vi "Accessories.vi"(11 "Full System Configuration":T2={"Rack"=enum."15U; 1-Phase; 16A; 100-240V", "Middle Rail"=enum."None", "Ballast"={"Main"=0, "Small"=0, "Side"=0}, "Front Panel I/O"={"EMO Button"=FALSE, "USB 3.0"=FALSE, "Display"=FALSE, "1st USB 2.0"=FALSE, "2nd USB 2.0"=FALSE, "Ethernet 3"=FALSE, "EMO Extension (3rd Party)"=FALSE, "EMO Extension (Rack In & Out)"=FALSE, "Aux Dual C13 QAC Outlets"=FALSE, "Residual-current Circuit Breaker"=FALSE, "Serial"=FALSE, "GPIB"=FALSE}, "Rear Panel I/O"={"Rear Panel I/O Configuration"=enum."Blank Panel", "EMO Button"=FALSE, "Power, Status & Banana Ground"=FALSE, "Ethernet 2"=FALSE, "Display"=FALSE, "USB 3.0"=FALSE, "DIO"=FALSE, "GPIB"=FALSE, "Aux Dual C13 QAC Outlets"=FALSE, "Residual-current Circuit Breaker"=FALSE, "Serial"=FALSE, "SMA"=FALSE}, "Miscellaneous Options"={"Eyebolts"=FALSE, "Tower Light"=FALSE, "Top/Side Monitor Mount Kit"=FALSE, "24\" Monitor"=FALSE, "Keyboard & Mouse"=FALSE, "Secondary Ethernet Switch"=FALSE, "Extra USB Hub"=FALSE, "USB-6509"=FALSE, "Front Door"=enum."38U (Solid) IG", "Primary Ethernet Switch"=enum."Item 0", "Use Posture"=enum."Item 0"}, "Accessories"={"Screw Type"=enum."10-32", "Cage Nuts & Screws"=0.0, "Filler Panel Color"=enum."Interface Gray", "1U"=0.0, "2U"=0.0, "3U"=0.0}} {"Ballast"."Side" max=5 step=1; "Ballast"."Small" max=5 step=1; "Ballast"."Main" max=5 step=1}) -> (3 "Accessories Out":T1[](array[typedef]))   [LabVIEW 2023]
uses:
  Option Type Defs/Full System Configuration.ctl
  Option Type Defs/Rack.ctl
  Option Type Defs/Middle Rail.ctl
  Option Type Defs/Ballast.ctl
  Option Type Defs/Front Panel IO.ctl
  Option Type Defs/Rear Panel IO.ctl
  Option Type Defs/Rear Panel IO Configuration.ctl
  Option Type Defs/Miscellaneous Options.ctl
  Option Type Defs/Front Door.ctl
  Option Type Defs/Accessories.ctl
  Option Type Defs/Screw Types.ctl
  Option Type Defs/Filler Panel Color.ctl
  Option Type Defs/Parts List.ctl
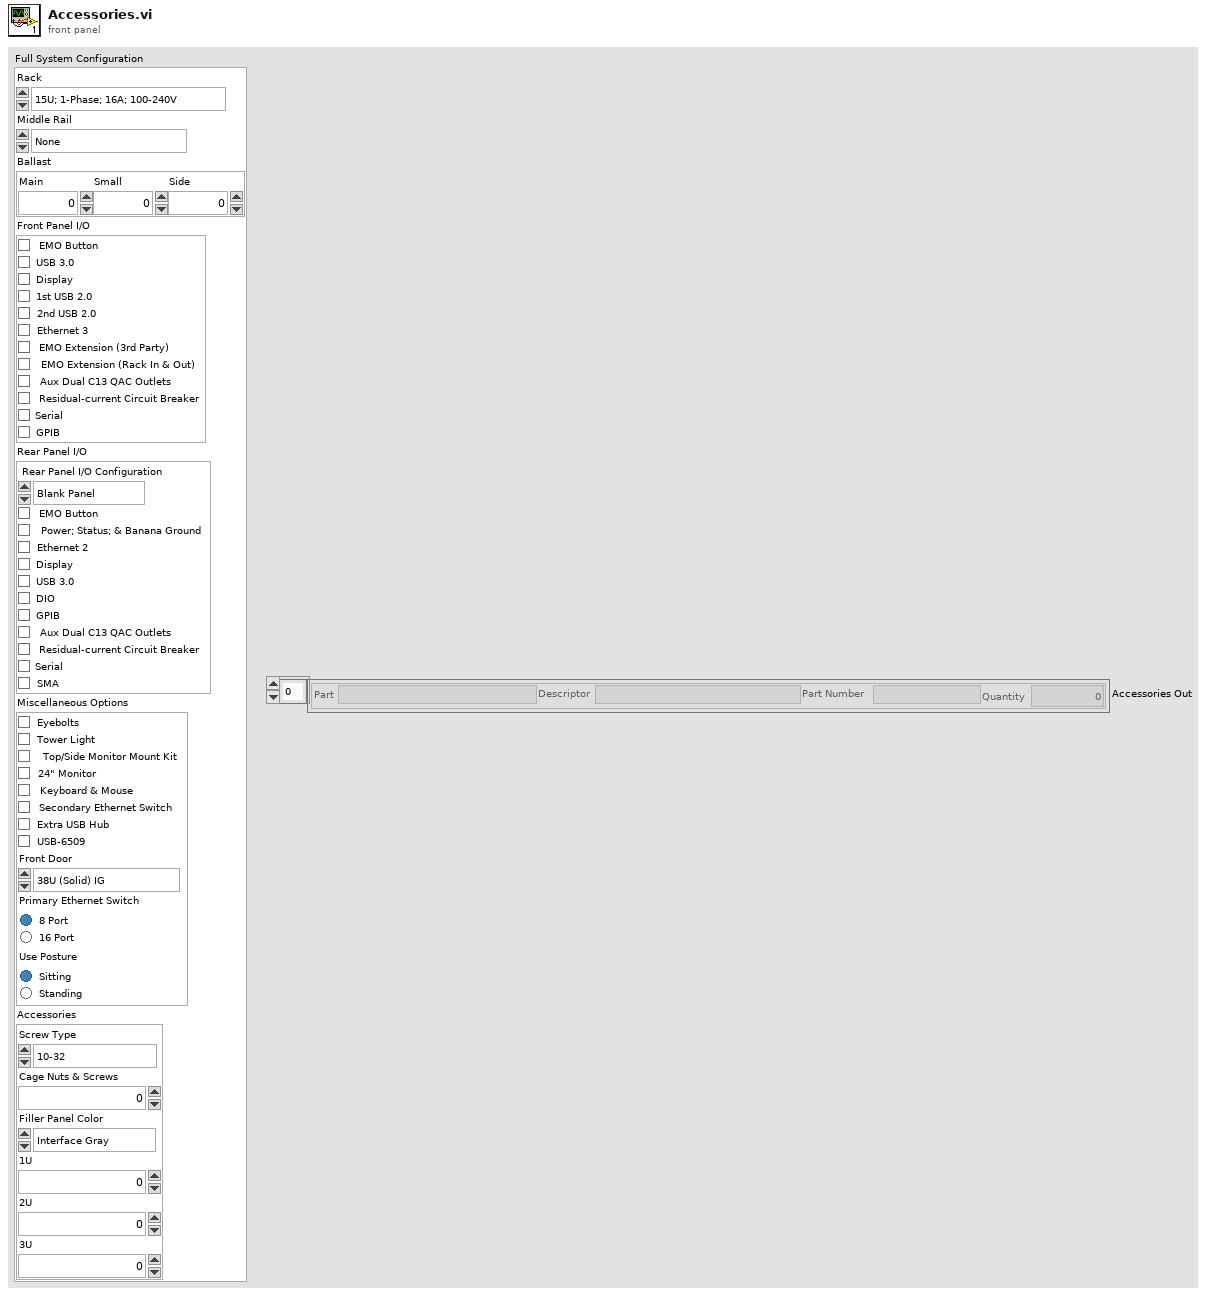
[diagram p1: front panel]
types:
  T1 = typedef "Parts List.ctl" = cluster{"Part":string, "Descriptor":string, "Part Number":string, "Quantity":dbl}
  T2 = typedef "Full System Configuration.ctl" = cluster{"Rack":T3, "Middle Rail":T4, "Ballast":T5, "Front Panel I/O":T6, "Rear Panel I/O":T7, "Miscellaneous Options":T9, "Accessories":T11}
  T3 = typedef "Rack.ctl" = enum16{"15U; 1-Phase; 16A; 100-240V", "15U; 1-Phase; 24A; 100-240V", "38U; 3-Phase Delta; 50A; 200-240V", "38U; 1-Phase; 24A; 100-120V", "38U; 3-Phase Wye; 50A; 200-240V", "38U; 3-Phase Delta; 50A; 380-480V", "38U; 3-Phase Delta; 32A; 200-240V", "38U; 3-Phase Wye; 16A; 100-240V", "44U; 1-Phase; 24A; 100-240V", "44U; 3-Phase Delta; 32A; 200-240V"}
  T4 = typedef "Middle Rail.ctl" = enum16{"None", "Flip Side Rear; D=168.83mm", "Parallel Rear; D=145mm", "Flip Side Front; D=145mm", "Parallel Front; D=145mm"}
  T5 = typedef "Ballast.ctl" = cluster{"Main":u16, "Small":u16, "Side":u16}
  T6 = typedef "Front Panel IO.ctl" = cluster{"EMO Button":bool, "USB 3.0":bool, "Display":bool, "1st USB 2.0":bool, "2nd USB 2.0":bool, "Ethernet 3":bool, "EMO Extension (3rd Party)":bool, "EMO Extension (Rack In & Out)":bool, "Aux Dual C13 QAC Outlets":bool, "Residual-current Circuit Breaker":bool, "Serial":bool, "GPIB":bool}
  T7 = typedef "Rear Panel IO.ctl" = cluster{"Rear Panel I/O Configuration":T8, "EMO Button":bool, "Power, Status & Banana Ground":bool, "Ethernet 2":bool, "Display":bool, "USB 3.0":bool, "DIO":bool, "GPIB":bool, "Aux Dual C13 QAC Outlets":bool, "Residual-current Circuit Breaker":bool, "Serial":bool, "SMA":bool}
  T8 = typedef "Rear Panel IO Configuration.ctl" = enum16{"Blank Panel", "Fully Populated Panel", "Custom Panel"}
  T9 = typedef "Miscellaneous Options.ctl" = cluster{"Eyebolts":bool, "Tower Light":bool, "Top/Side Monitor Mount Kit":bool, "24\" Monitor":bool, "Keyboard & Mouse":bool, "Secondary Ethernet Switch":bool, "Extra USB Hub":bool, "USB-6509":bool, "Front Door":T10, "Primary Ethernet Switch":enum32{"Item 0", "Item 1"}, "Use Posture":enum32{"Item 0", "Item 1"}}
  T10 = typedef "Front Door.ctl" = enum16{"None", "38U (Solid) IG", "38U (Solid) EG", "38U: Top 14U (Solid) IG", "38U (Clear) IG", "44U (Solid) IG", "44U (Solid) EG"}
  T11 = typedef "Accessories.ctl" = cluster{"Screw Type":T12, "Cage Nuts & Screws":dbl, "Filler Panel Color":T13, "1U":dbl, "2U":dbl, "3U":dbl}
  T12 = typedef "Screw Types.ctl" = enum16{"None", "M6 (Most Common)", "10-32", "12-24"}
  T13 = typedef "Filler Panel Color.ctl" = enum16{"None", "Interface Gray", "Environmental Gray"}
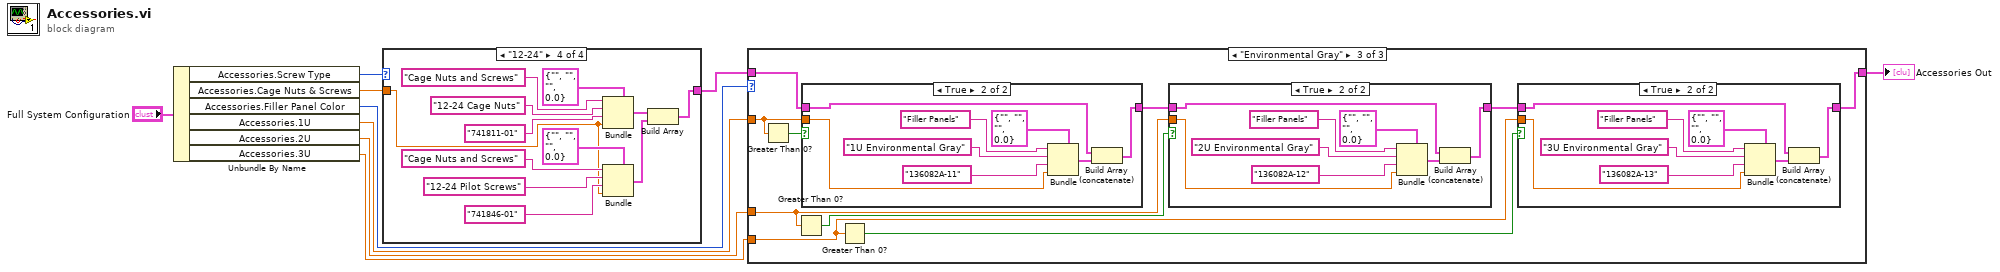
[diagram p0: block diagram]
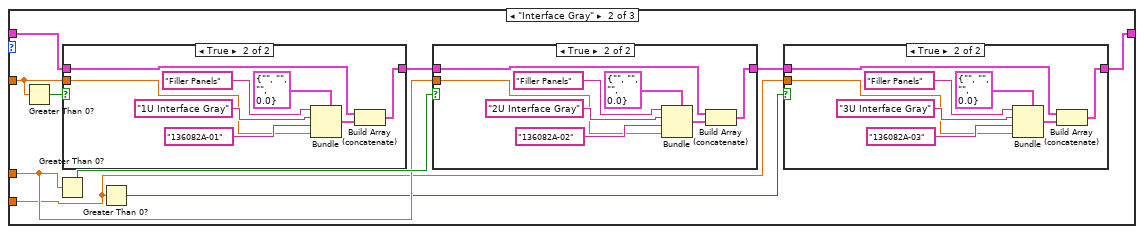
[diagram p3: hidden frame]
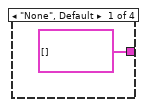
[diagram p10: hidden frame]
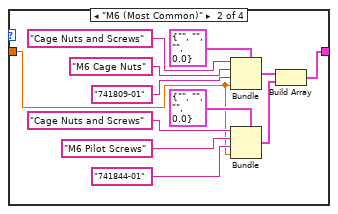
[diagram p11: hidden frame]
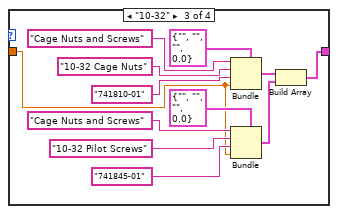
[diagram p12: hidden frame]
diagram:
  n1 = Unbundle By Name("Full System Configuration") -> ("Accessories.Screw Type"=w8:T12, "Accessories.Cage Nuts & Screws"=w7:dbl, "Accessories.Filler Panel Color"=w6:T13, "Accessories.1U"=w4:dbl, "Accessories.2U"=w3:dbl, "Accessories.3U"=w2:dbl)
  n2 = case shown="\"12-24\"" w8 {
    tunnel: [T1[] [] ("cluster") w12 w24 w36] -> w5
    tunnel: w7 -> [_ w11 w23 w35]
    frame "None", Default {
    }
    frame "M6 (Most Common)" {
      n3 = Bundle(cluster=T1 {"Part"="", "Descriptor"="", "Part Number"="", "Quantity"=0.0}, "Part"="Cage Nuts and Screws", "Descriptor"="M6 Cage Nuts", "Part Number"="741809-01", "Quantity"=w11) -> (w14:T1)
      n4 = Bundle(cluster=T1 {"Part"="", "Descriptor"="", "Part Number"="", "Quantity"=0.0}, "Part"="Cage Nuts and Screws", "Descriptor"="M6 Pilot Screws", "Part Number"="741844-01", "Quantity"=w11) -> (w13:T1)
      n5 = Build Array(w14, w13) -> (w12:T1[])
    }
    frame "10-32" {
      n6 = Bundle(cluster=T1 {"Part"="", "Descriptor"="", "Part Number"="", "Quantity"=0.0}, "Part"="Cage Nuts and Screws", "Descriptor"="10-32 Cage Nuts", "Part Number"="741810-01", "Quantity"=w23) -> (w26:T1)
      n7 = Bundle(cluster=T1 {"Part"="", "Descriptor"="", "Part Number"="", "Quantity"=0.0}, "Part"="Cage Nuts and Screws", "Descriptor"="10-32 Pilot Screws", "Part Number"="741845-01", "Quantity"=w23) -> (w25:T1)
      n8 = Build Array(w26, w25) -> (w24:T1[])
    }
    frame "12-24" {
      n9 = Bundle(cluster=T1 {"Part"="", "Descriptor"="", "Part Number"="", "Quantity"=0.0}, "Part"="Cage Nuts and Screws", "Descriptor"="12-24 Cage Nuts", "Part Number"="741811-01", "Quantity"=w35) -> (w38:T1)
      n10 = Bundle(cluster=T1 {"Part"="", "Descriptor"="", "Part Number"="", "Quantity"=0.0}, "Part"="Cage Nuts and Screws", "Descriptor"="12-24 Pilot Screws", "Part Number"="741846-01", "Quantity"=w35) -> (w37:T1)
      n11 = Build Array(w38, w37) -> (w36:T1[])
    }
  }
  n12 = case shown="\"Environmental Gray\"" w6 {
    tunnel: w5 -> [w47 w57 w94]
    tunnel: w4 -> [_ w55 w92]
    tunnel: [w47 w48 w85] -> w1
    tunnel: w3 -> [_ w53 w90]
    tunnel: w2 -> [_ w50 w87]
    frame "None", Default {
    }
    frame "Interface Gray" {
      n13 = Greater Than 0?(x=w55) -> (x > 0?=w56:bool)
      n14 = Greater Than 0?(x=w53) -> (x > 0?=w54:bool)
      n15 = case shown="True" w56 {
        tunnel: w57 -> [w76 w80]
        tunnel: [w76 w78] -> w52
        tunnel: w55 -> [_ w77]
        frame False {
        }
        frame True {
          n16 = Bundle(cluster=T1 {"Part"="", "Descriptor"="", "Part Number"="", "Quantity"=0.0}, "Part"="Filler Panels", "Descriptor"="1U Interface Gray", "Part Number"="136082A-01", "Quantity"=w77) -> (w79:T1)
          n17 = Build Array (concatenate)(w80, w79) -> (w78:T1[])
        }
      }
      n18 = Greater Than 0?(x=w50) -> (x > 0?=w49:bool)
      n19 = case shown="True" w54 {
        tunnel: w52 -> [w67 w71]
        tunnel: [w67 w69] -> w51
        tunnel: w53 -> [_ w68]
        frame False {
        }
        frame True {
          n20 = Bundle(cluster=T1 {"Part"="", "Descriptor"="", "Part Number"="", "Quantity"=0.0}, "Part"="Filler Panels", "Descriptor"="2U Interface Gray", "Part Number"="136082A-02", "Quantity"=w68) -> (w70:T1)
          n21 = Build Array (concatenate)(w71, w70) -> (w69:T1[])
        }
      }
      n22 = case shown="True" w49 {
        tunnel: w51 -> [w58 w62]
        tunnel: [w58 w60] -> w48
        tunnel: w50 -> [_ w59]
        frame False {
        }
        frame True {
          n23 = Bundle(cluster=T1 {"Part"="", "Descriptor"="", "Part Number"="", "Quantity"=0.0}, "Part"="Filler Panels", "Descriptor"="3U Interface Gray", "Part Number"="136082A-03", "Quantity"=w59) -> (w61:T1)
          n24 = Build Array (concatenate)(w62, w61) -> (w60:T1[])
        }
      }
    }
    frame "Environmental Gray" {
      n25 = Greater Than 0?(x=w92) -> (x > 0?=w93:bool)
      n26 = Greater Than 0?(x=w90) -> (x > 0?=w91:bool)
      n27 = case shown="True" w93 {
        tunnel: w94 -> [w113 w117]
        tunnel: [w113 w115] -> w89
        tunnel: w92 -> [_ w114]
        frame False {
        }
        frame True {
          n28 = Bundle(cluster=T1 {"Part"="", "Descriptor"="", "Part Number"="", "Quantity"=0.0}, "Part"="Filler Panels", "Descriptor"="1U Environmental Gray", "Part Number"="136082A-11", "Quantity"=w114) -> (w116:T1)
          n29 = Build Array (concatenate)(w117, w116) -> (w115:T1[])
        }
      }
      n30 = Greater Than 0?(x=w87) -> (x > 0?=w86:bool)
      n31 = case shown="True" w91 {
        tunnel: w89 -> [w104 w108]
        tunnel: [w104 w106] -> w88
        tunnel: w90 -> [_ w105]
        frame False {
        }
        frame True {
          n32 = Bundle(cluster=T1 {"Part"="", "Descriptor"="", "Part Number"="", "Quantity"=0.0}, "Part"="Filler Panels", "Descriptor"="2U Environmental Gray", "Part Number"="136082A-12", "Quantity"=w105) -> (w107:T1)
          n33 = Build Array (concatenate)(w108, w107) -> (w106:T1[])
        }
      }
      n34 = case shown="True" w86 {
        tunnel: w88 -> [w95 w99]
        tunnel: [w95 w97] -> w85
        tunnel: w87 -> [_ w96]
        frame False {
        }
        frame True {
          n35 = Bundle(cluster=T1 {"Part"="", "Descriptor"="", "Part Number"="", "Quantity"=0.0}, "Part"="Filler Panels", "Descriptor"="3U Environmental Gray", "Part Number"="136082A-13", "Quantity"=w96) -> (w98:T1)
          n36 = Build Array (concatenate)(w99, w98) -> (w97:T1[])
        }
      }
    }
  }
  "Accessories Out" <- w1
